vi "Initialize Gantry.vi"(7 "Console Log in":refnum<class "Console Log.lvclass">, 8 "error in (no error)":errorcluster, 9 "Virtual Mode":T1, 10 "Prompt for Virtual Mode":bool, 11 "gScript Interpreter in":refnum<class "gScript Interpreter.lvclass">) -> (0 "error out":errorcluster, 2 "Gantry out":refnum<class "Gantry.lvclass">, 3 "gScript Interpreter out":refnum<class "gScript Interpreter.lvclass">, 5 "Console Log out":refnum<class "Console Log.lvclass">)   [LabVIEW 2023, in "gScript Interpreter.lvclass"]
uses:
  gScript Interpreter.lvclass
  Application Utilities/Console Log/Console Log.lvclass
  Shared Components/Gantry Class/Gantry.lvclass
  Shared Components/Gantry Class/Type Definitions/Virtual Modes.ctl
  Shared Components/Gantry Class/Type Definitions/Init_Modes.ctl
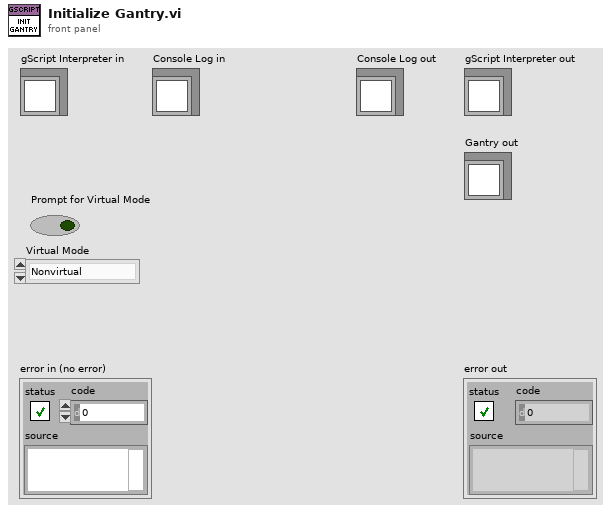
[diagram p1: front panel]
types:
  T1 = typedef "Virtual Modes.ctl" = enum16{"Nonvirtual", "Virtual"}
  T2 = typedef "Init_Modes.ctl" = enum16{"Full", "Robot Only", "Dispenser Only", "Cameras Only", "Robot and Cameras", "Robot and Cameras and Dispenser", "Manifold Only"}
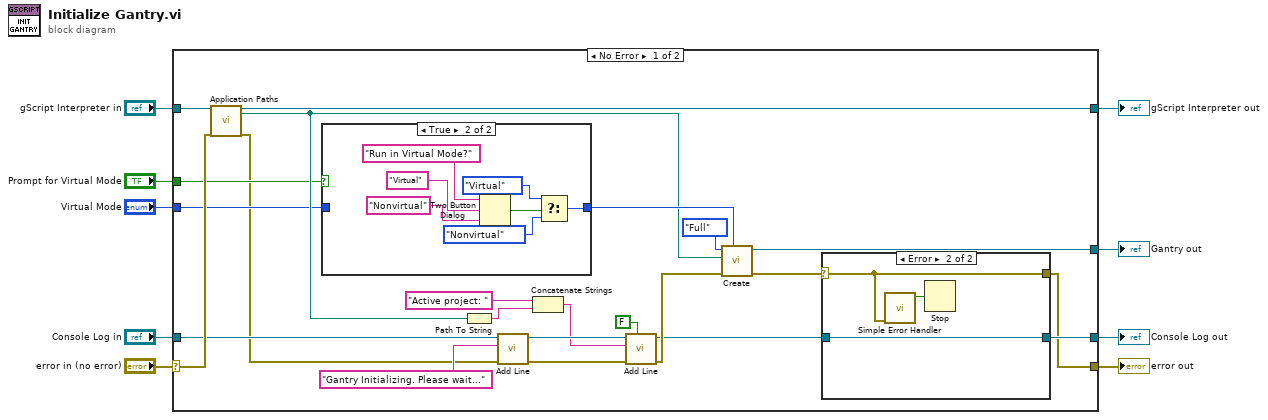
[diagram p0: block diagram]
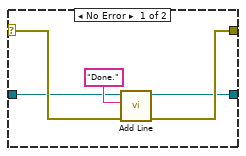
[diagram p2: hidden frame]
diagram:
  n1 = case shown="No Error" "error in (no error)" {
    selector: "error in (no error)" -> [w20 w51]
    tunnel: [w12 w51] -> w8
    tunnel: [w18 w50] -> w6
    tunnel: "gScript Interpreter in" -> [w19 w50]
    tunnel: [w21 _] -> w5
    tunnel: [w13 w49] -> w4
    tunnel: "Console Log in" -> [w11 w49]
    tunnel: "Prompt for Virtual Mode" -> [w17 _]
    tunnel: "Virtual Mode" -> [w16 _]
    frame No Error {
      n2 = call "Application Paths.vi"("gScript Interpreter in"=w19, "error in (no error)"=w20) -> ("gScript Interpreter out"=w18:refnum<class "gScript Interpreter.lvclass">, "Project Path"=w22:path, "error out"=w10:errorcluster)  [unwired: 12 in, 3 out]
      n3 = case shown="True" w17 {
        tunnel: [w41 w43] -> w30
        tunnel: w16 -> [w41 _]
        frame False {
        }
        frame True {
          n4 = Two Button Dialog(message="Run in Virtual Mode?", 1:"Nonvirtual" ("F button name (\"Cancel\")"), 2:"Virtual" ("T button name (\"OK\")")) -> (T button?=w42:bool)
          n5 = Select(t=Virtual_Modes."Virtual" ("Virtual Mode"), s=w42, f=Virtual_Modes."Nonvirtual" ("Virtual Mode")) -> (s? t:f=w43:T1)
        }
      }
      n6 = Path To String(path=w22) -> (string=w25:string)
      n7 = call "Add Line.vi"("error in"=w10, "String"="Gantry Initializing. Please wait...", "Console Log in"=w11) -> ("error out"=w24:errorcluster, "Console Log out"=w29:refnum<class "Console Log.lvclass">)  [unwired: 7 in]
      n8 = Concatenate Strings("Active project: " ("format string"), w25) -> (w28:string)
      n9 = call "Add Line.vi"("Timestamp"=FALSE, "error in"=w24, "String"=w28, "Console Log in"=w29) -> ("error out"=w23:errorcluster, "Console Log out"=w15:refnum<class "Console Log.lvclass">)  [unwired: 6 in]
      n10 = call "Create.vi"("Virtual Mode"=w30, "error in"=w23, "Project Path"=w22, "Init Mode"=Init_Modes."Full") -> ("error out"=w14:errorcluster, "Gantry out"=w21:refnum<class "Gantry.lvclass">)  [unwired: 6 in]
      n11 = case shown="Error" w14 {
        selector: w14 -> [w37 w40]
        tunnel: [w36 w40] -> w12
        tunnel: w15 -> [w34 w38]
        tunnel: [w33 w38] -> w13
        frame No Error {
          n12 = call "Add Line.vi"("error in"=w37, "String"="Done.", "Console Log in"=w34) -> ("error out"=w36:errorcluster, "Console Log out"=w33:refnum<class "Console Log.lvclass">)  [unwired: 7 in]
        }
        frame Error {
          n13 = call <vilib>:"Simple Error Handler.vi"("error in (no error)"=w40) -> ("error?"=w39:bool)  [unwired: 4 in, 4 out]
          n14 = Stop(stop? (T)=w39) -> ()
        }
      }
    }
    frame Error {
    }
  }
  "error out" <- w8
  "gScript Interpreter out" <- w6
  "Console Log out" <- w4
  "Gantry out" <- w5
